vi "_Remote Connect.vi"(4 "error in (no error)":errorcluster) -> (0 "error out":errorcluster, 3 "TCP":bool)   [LabVIEW 2015]
uses:
  Types/_RT Command.ctl
  Global Parameters.vi
panel:
  out "Info":string
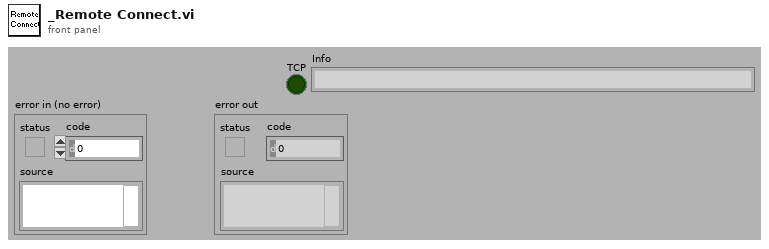
[diagram p1: front panel]
types:
  T1 = typedef "_RT Command.ctl" = enum16{"xml Start Run", "xml Start Actual Run", "xml Stop Run", "xml Runtime Update", "xml Get Status", "xml Get Table", "xml Set Table", "xml Get Configuration", "xml System Status", "xml Set LC Input Logic", "xml Get Data", "xml Get Info", "Start", "StartActualRun", "Stop", "Runtime Update", "Get Data", "Get Info", "Get Status", "Get Param", "Get Config", "Get Table", "Read ADC", "Set Oscillator", "Update Config", "Update Table", "Set All Pol", "Set Pol and DC", "Set Max Mass", "Toggle RP", "Toggle EL", "Set PIC", "Initialize Turbo", "Send Turbo Comm", "Close Turbo", "P1", "P2", "P3", "Send Serial", "Set LC Out", "Get LC In", "Read VAC", "Test Table", "Toggle Power", "Get Startup", "Set Startup", "Get ADC Table", "Set ADC Table", "Get Brief Status", "Get Detail Status", "Auxiliary Update", "Set CC Logics", "Set CC Input Logics", "Ignore Error", "invalid"}
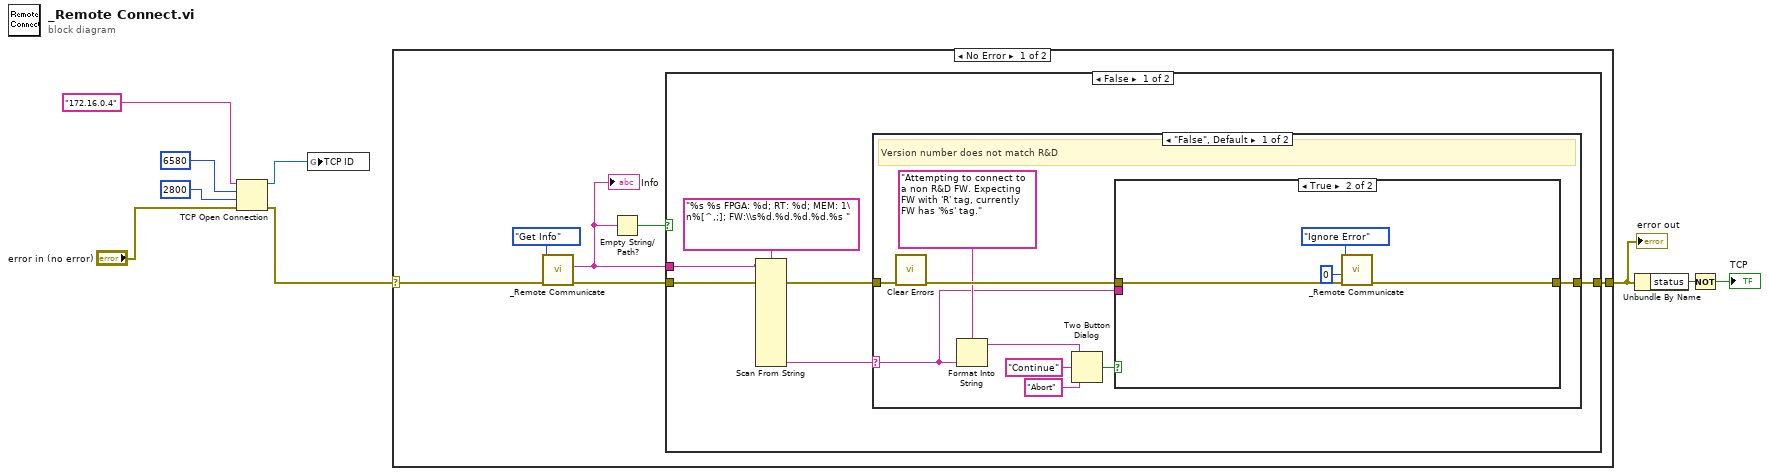
[diagram p0: block diagram]
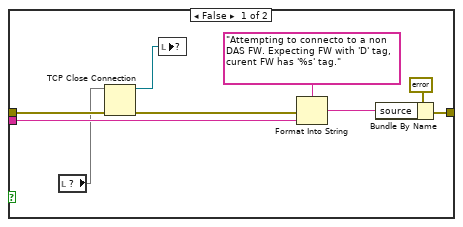
[diagram p2: hidden frame]
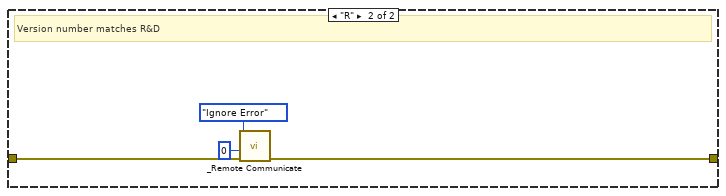
[diagram p3: hidden frame]
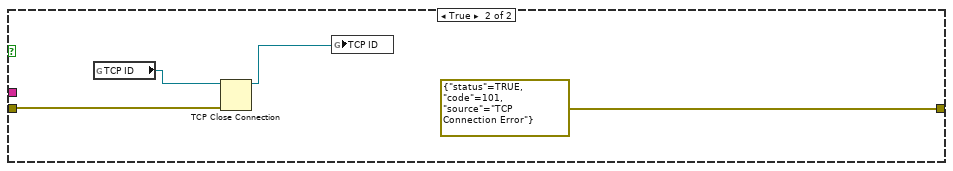
[diagram p4: hidden frame]
diagram:
  n1 = TCP Open Connection(address="172.16.0.4" ("IP Address"), remote port or service name=u16 6580 ("remote port"), timeout ms (60000)=2800, error in (no error)="error in (no error)") -> (connection ID=w1:refnum<k5>, error out=w2:errorcluster)  [unwired: 1 out]
  n2 = global write "Global Parameters.vi" "TCP ID"(w1) -> ()
  n3 = case shown="No Error" w2 {
    selector: w2 -> [w10 w52]
    tunnel: [w13 w52] -> w8
    frame No Error {
      n4 = call "_Remote Communicate.vi"("error in (no error)"=w10, "Command"=_RT_Command."Get Info") -> ("error out"=w14:errorcluster, "Info"=w11:string)  [unwired: 4 in, 2 out]
      "Info" <- w11
      n5 = Empty String/Path?(string/path=w11) -> (empty?=w12:bool)
      n6 = case shown="False" w12 {
        tunnel: w14 -> [w19 w50]
        tunnel: [w21 errorcluster {"status"=TRUE, "code"=101, "source"="TCP Connection Error"} ("error out")] -> w13
        tunnel: w11 -> [w16 _]
        frame False {
          n7 = Scan From String(format string="%s %s FPGA: %d; RT: %d; MEM: 1\n%[^,;]; FW:\\s%d.%d.%d.%d.%s ", input string=w16, error in=w19) -> (error out=w18:errorcluster, output 10=w17:string)  [unwired: 20 in, 2 out]
          n8 = case shown="\"False\", Default" w17 {
            selector: w17 -> [w22 _]
            tunnel: [w25 w45] -> w21
            tunnel: w18 -> [w30 w44]
            frame "False", Default {
              # "Version number does not match R&D"
              n9 = call <vilib>:"Clear Errors.vi"("error in (no error)"=w30) -> ("error out"=w26:errorcluster)  [unwired: 5 in, 1 out]
              n10 = Format Into String(format string="Attempting to connect to a non R&D FW. Expecting FW with 'R' tag, currently FW has '%s' tag." ("message"), w22) -> (resulting string=w23:string)  [unwired: 2 in, 1 out]
              n11 = Two Button Dialog(message=w23, 1:"Abort" ("F button name (\"Cancel\")"), 2:"Continue" ("T button name (\"OK\")")) -> (T button?=w27:bool)
              n12 = case shown="True" w27 {
                tunnel: w26 -> [w39 w40]
                tunnel: [w33 w41] -> w25
                tunnel: w22 -> [w35 _]
                frame False {
                  n13 = local read item#-1() -> (w31)
                  n14 = TCP Close Connection(connection ID=w31, error in (no error)=w39) -> (connection ID out=w32:refnum<k5>, error out=w34:errorcluster)  [unwired: 1 in]
                  n15 = local write item#-1(w32) -> ()
                  n16 = Format Into String(format string="Attempting to connecto to a non DAS FW. Expecting FW with 'D' tag, curent FW has '%s' tag." ("source"), error in=w34, w35) -> (resulting string=w36:string)  [unwired: 1 in, 1 out]
                  n17 = Bundle By Name(cluster=errorcluster {"status"=TRUE, "code"=110, "source"="Attempting to connecto to a non MD FW"} ("error out"), "source"=w36) -> (w33:errorcluster)
                }
                frame True {
                  n18 = call "_Remote Communicate.vi"("error in (no error)"=w40, "DC Param"=u16 0, "Command"=_RT_Command."Ignore Error") -> ("error out"=w41:errorcluster)  [unwired: 3 in, 3 out]
                }
              }
            }
            frame "R" {
              # "Version number matches R&D"
              n19 = call "_Remote Communicate.vi"("error in (no error)"=w44, "DC Param"=u16 0, "Command"=_RT_Command."Ignore Error") -> ("error out"=w45:errorcluster)  [unwired: 3 in, 3 out]
            }
          }
        }
        frame True {
          n20 = global read "Global Parameters.vi" "TCP ID"() -> (w48:refnum<k5>)
          n21 = TCP Close Connection(connection ID=w48, error in (no error)=w50) -> (connection ID out=w49:refnum<k5>)  [unwired: 1 in, 1 out]
          n22 = global write "Global Parameters.vi" "TCP ID"(w49) -> ()
        }
      }
    }
    frame Error {
    }
  }
  "error out" <- w8
  n23 = Unbundle By Name(w8) -> ("status"=w9:bool)
  n24 = Not(x=w9) -> (.not. x?=→"TCP":bool)
